vi "validate key value pair.vi"(8 "error in":errorcluster, 9 "value":string, 10 "key":string, 11 "WaveformAcq configuration in":refnum<class "WaveformAcq configuration.lvclass">) -> (0 "error out":errorcluster, 3 "WaveformAcq configuration out":refnum<class "WaveformAcq configuration.lvclass">)   [LabVIEW 2017, in "WaveformAcq configuration.lvclass"]
uses:
  WaveformAcq configuration.lvclass
  <vilib>/NI/DCAF/Tag Editor Core/control module/configuration/control module configuration.lvclass
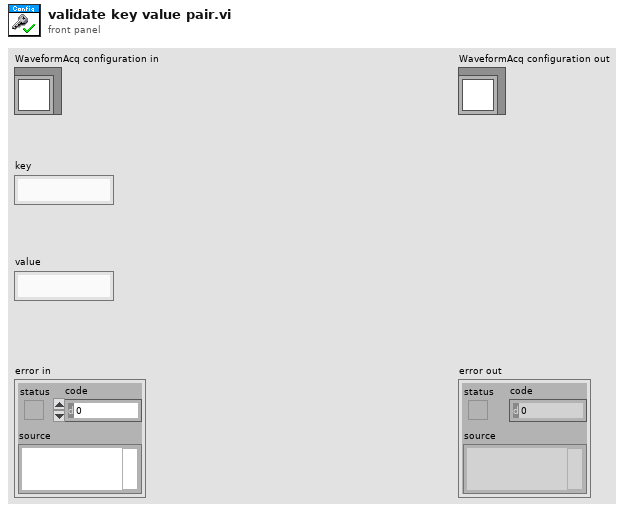
[diagram p1: front panel]
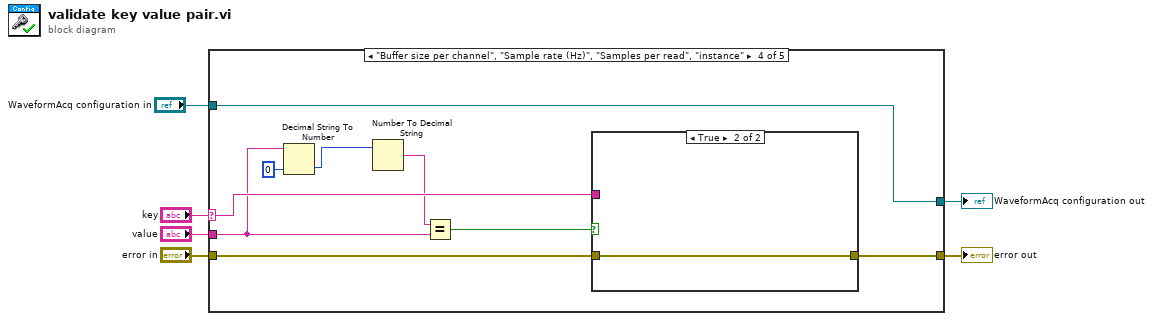
[diagram p0: block diagram]
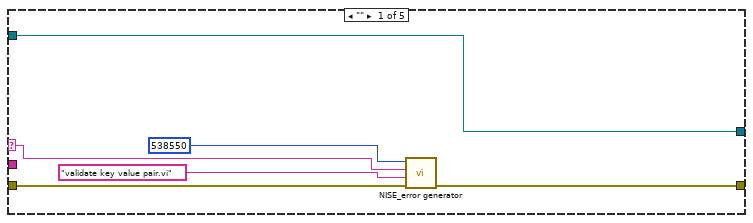
[diagram p2: hidden frame]
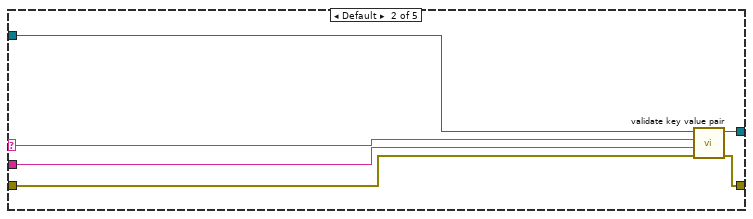
[diagram p3: hidden frame]
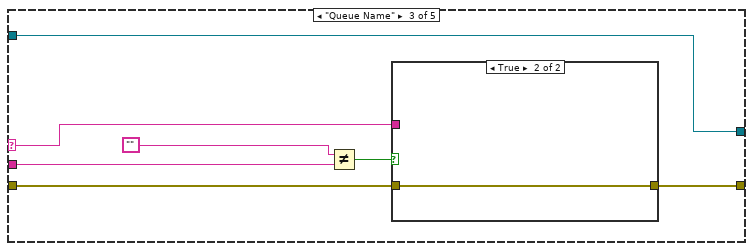
[diagram p4: hidden frame]
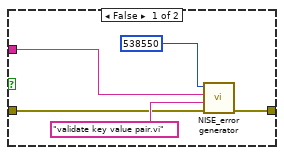
[diagram p5: hidden frame]
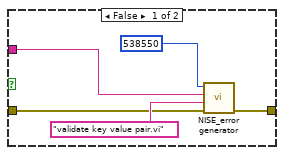
[diagram p6: hidden frame]
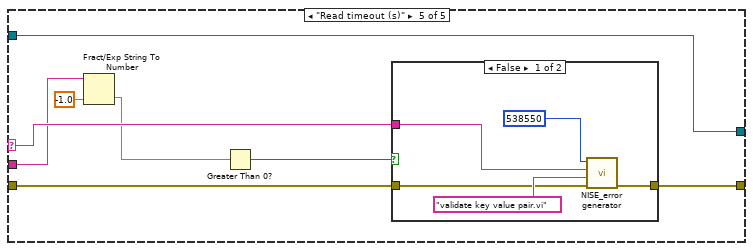
[diagram p7: hidden frame]
diagram:
  n1 = case shown="\"Buffer size per channel\", \"Sample rate (Hz)\", \"Samples per read\", \"instance\"" "key" {
    selector: "key" -> [w9 w13 w23 w40 w54]
    tunnel: [w7 w18 w21 w38 w52] -> w6
    tunnel: [w12 w17 w20 w37 w51] -> w5
    tunnel: "error in" -> [w8 w16 w22 w39 w53]
    tunnel: "value" -> [_ w15 w25 w33 w50]
    tunnel: "WaveformAcq configuration in" -> [w12 w14 w20 w37 w51]
    frame "" {
      n2 = call <vilib>:"NISE_error generator.vi"("error in"=w8, "source"="validate key value pair.vi", "append error message"=w9, "error code (0)"=538550) -> ("error out"=w7:errorcluster)  [unwired: 5 in]
    }
    frame Default {
      n3 = call-parent "validate key value pair.vi"("error in"=w16, "value"=w15, "key"=w13, "fixed channel configuration in"=w14) -> ("error out"=w18:errorcluster, "fixed channel configuration out"=w17:refnum<class "WaveformAcq configuration.lvclass">)  [unwired: 6 in]
    }
    frame "Queue Name" {
      n4 = Not Equal?(x="", y=w25) -> (x != y?=w19:bool)
      n5 = case shown="True" w19 {
        tunnel: w23 -> [w28 _]
        tunnel: w22 -> [w27 w31]
        tunnel: [w26 w31] -> w21
        frame False {
          n6 = call <vilib>:"NISE_error generator.vi"("error in"=w27, "source"="validate key value pair.vi", "append error message"=w28, "error code (0)"=538550) -> ("error out"=w26:errorcluster)  [unwired: 5 in]
        }
        frame True {
        }
      }
    }
    frame "Buffer size per channel", "Sample rate (Hz)", "Samples per read", "instance" {
      n7 = Decimal String To Number(string=w33, default (0L)=u32 0 ("default (0 I32)")) -> (number=w35:u32)  [unwired: 1 in, 1 out]
      n8 = Number To Decimal String(number=w35) -> (decimal integer string=w34:string)  [unwired: 1 in]
      n9 = Equal?(x=w34, y=w33) -> (x = y?=w32:bool)
      n10 = case shown="True" w32 {
        tunnel: w40 -> [w43 _]
        tunnel: w39 -> [w42 w46]
        tunnel: [w41 w46] -> w38
        frame False {
          n11 = call <vilib>:"NISE_error generator.vi"("error in"=w42, "source"="validate key value pair.vi", "append error message"=w43, "error code (0)"=538550) -> ("error out"=w41:errorcluster)  [unwired: 5 in]
        }
        frame True {
        }
      }
    }
    frame "Read timeout (s)" {
      n12 = Fract/Exp String To Number(string=w50, default (0 dbl)=-1.0 ("default (0 DBL)")) -> (number=w47:dbl)  [unwired: 2 in, 1 out]
      n13 = Greater Than 0?(x=w47) -> (x > 0?=w49:bool)
      n14 = case shown="False" w49 {
        tunnel: w54 -> [w57 _]
        tunnel: w53 -> [w56 w60]
        tunnel: [w55 w60] -> w52
        frame False {
          n15 = call <vilib>:"NISE_error generator.vi"("error in"=w56, "source"="validate key value pair.vi", "append error message"=w57, "error code (0)"=538550) -> ("error out"=w55:errorcluster)  [unwired: 5 in]
        }
        frame True {
        }
      }
    }
  }
  "error out" <- w6
  "WaveformAcq configuration out" <- w5
